vi "main_image_aquisition.vi"(5 "notifier in":refnum<notifier>, 6 "error in (no error)":errorcluster, 8 "queue in":refnum<queue>, 9 "Session In":T1) -> (0 "error out":errorcluster)   [LabVIEW 2019]
uses:
  <vilib>/userdefined/High Color/IMAQdx.ctl
  <vilib>/vision/driver/IMAQdx.llb/IMAQdx Buffer Number Mode.ctl
  TimestampsFunctionalGlobalOperations.ctl
  ParametersGlobal.vi
  DebugGlobal.vi
  <vilib>/vision/driver/NI_Vision_Acquisition_Software.lvlib
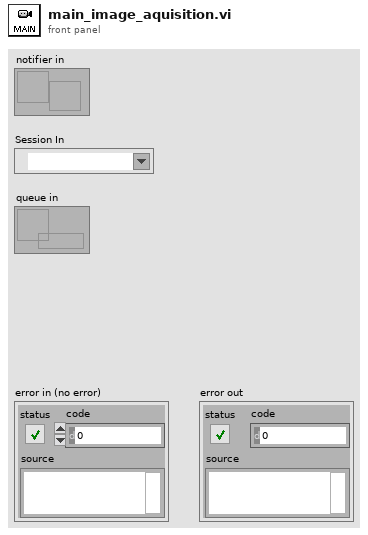
[diagram p1: front panel]
types:
  T1 = typedef "IMAQdx.ctl" = refnum<k21>
  T2 = typedef "Image Type" = u32
  T3 = typedef "IMAQ Image.ctl" = refnum<image>
  T4 = typedef "TimestampsFunctionalGlobalOperations.ctl" = enum16{"Initialize", "Dump", "UpdateTime", "ReadTime"}
  T5 = typedef "NI_Vision_Acquisition_Software.lvlib/IMAQdx Buffer Number Mode.ctl" = enum32{"Next", "Last", "Buffer Number", "Every", "Last New"}
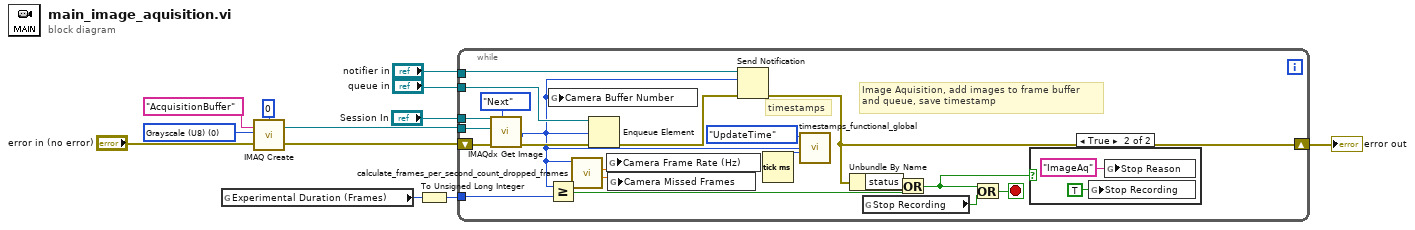
[diagram p0: block diagram]
diagram:
  w7 = T2 0 items=["Grayscale (U8)", "Grayscale (I16)", "Grayscale (SGL)", "Complex (CSG)", "RGB (U32)", "HSL (U32)", "RGB (U64)"] ("Image Type")
  n1 = global read "ParametersGlobal.vi" "Experimental Duration (Frames)"() -> (w2:i32)
  n2 = call "IMAQ Create"("Border Size"=0, "Image Name"="AcquisitionBuffer", "Image Type"=w7, "error in (no error)"="error in (no error)") -> ("New Image"=w5:T3, "error out"=w3:errorcluster)  [unwired: 1 in]
  n3 = To Unsigned Long Integer(number=w2) -> (unsigned 32bit integer=w1:u32)
  n4 = while {
    tunnel: "queue in" -> [w30]
    tunnel: w5 -> [w29]
    tunnel: "Session In" -> [w28]
    shift-right: [w24] -> w9
    shift-left: w3 -> [w27]
    tunnel: "notifier in" -> [w25]
    tunnel: w1 -> [w23]
    stop <- w32 stop-if-true
    # "timestamps"
    # "Image Aquisition, add images to frame buffer\nand queue, save timestamp"
    n5 = call <vilib>:"IMAQdx Get Image.vi"("Buffer Number Mode (Next)"=IMAQdx_Buffer_Number_Mode."Next", "error in"=w27, "Image In"=w29, "Session In"=w28) -> ("error out"=w26:errorcluster, "Buffer Number Out"=w17:u32)  [unwired: 4 in, 2 out]
    n6 = Greater Or Equal?(x=w17, y=w23) -> (x >= y?=w21:bool)
    n7 = global write "DebugGlobal.vi" "Camera Buffer Number"(w17) -> ()
    n8 = call "calculate_frames_per_second_count_dropped_frames.vi"("Buffer Number"=w17) -> ("Missed Frames"=w15:dbl, "Processed Frames/s"=w16:dbl)  [unwired: 8 in, 1 out]
    n9 = Enqueue Element(queue=w30, element=w17, error in (no error)=w26) -> (error out=w18:errorcluster)  [unwired: 1 in, 2 out]
    n10 = global write "DebugGlobal.vi" "Camera Frame Rate (Hz)"(w16) -> ()
    n11 = global write "DebugGlobal.vi" "Camera Missed Frames"(w15) -> ()
    n12 = Send Notification(notification=w17, notifier=w25, error in (no error)=w18) -> (error out=w24:errorcluster)  [unwired: 1 out]
    n13 = Tick Count (ms)() -> (millisecond timer value=w19:u32)
    n14 = call "timestamps_functional_global.vi"("Timestamp In"=w19, "Buffer Number"=w17, "Operation"=TimestampsFunctionalGlobalOperations."UpdateTime") -> ()  [unwired: 2 in, 3 out]
    n15 = Unbundle By Name(w24) -> ("status"=w22:bool)
    n16 = global read "DebugGlobal.vi" "Stop Recording"() -> (w14:bool)
    n17 = Or(x=w22, y=w21) -> (x .or. y?=w20:bool)
    n18 = Or(x=w20, y=w14) -> (x .or. y?=w32:bool)
    n19 = case shown="True" w20 {
      frame False {
      }
      frame True {
        n20 = global write "DebugGlobal.vi" "Stop Recording"(TRUE ("stop")) -> ()
        n21 = global write "DebugGlobal.vi" "Stop Reason"("ImageAq" ("Stop Debug")) -> ()
      }
    }
  }
  "error out" <- w9
